vi "Init.vi"(8 "error in":errorcluster, 9 "IDNStr Override":string, 10 "Alias":string) -> (0 "error out":errorcluster, 3 "Instrument out":refnum<class "Instrument.lvclass">)   [LabVIEW 2014, in "Instrument.lvclass"]
uses:
  Instrument.lvclass
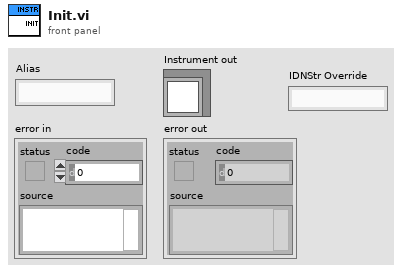
[diagram p1: front panel]
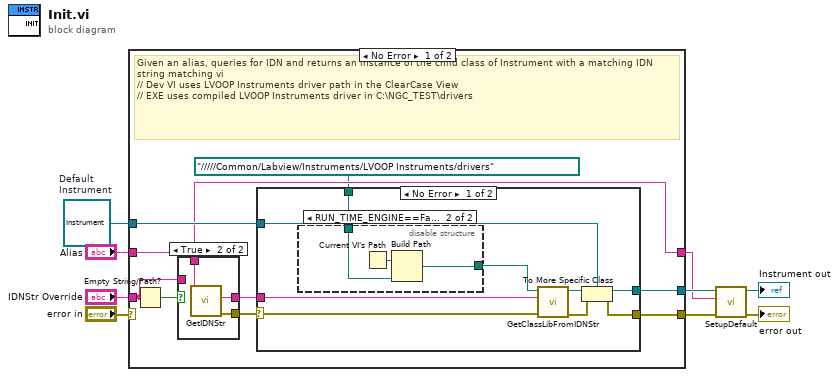
[diagram p0: block diagram]
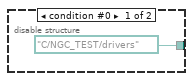
[diagram p3: hidden frame]
diagram:
  w7 = refnum<class "Instrument.lvclass"> refnum  # Default Instrument
  n1 = case shown="No Error" "error in" {
    selector: "error in" -> [_ w40]
    tunnel: "Alias" -> [w13 w38]
    tunnel: [w17 w39] -> w6
    tunnel: [w18 w40] -> w5
    tunnel: w7 -> [w14 w39]
    tunnel: [w13 w38] -> w2
    tunnel: "IDNStr Override" -> [w11 _]
    frame No Error {
      # "Given an alias, queries for IDN and returns an instance of the child class of Instrument with a matching IDN string matching vi\n// Dev VI uses LVOOP Instruments driver path in the ClearCase View\n// EXE uses compiled LVOOP Instruments driver in C:\\NGC_TEST\\drivers"
      n2 = Empty String/Path?(string/path=w11) -> (empty?=w12:bool)
      n3 = case shown="True" w12 {
        tunnel: [_ w22] -> w16
        tunnel: [w19 w21] -> w15
        tunnel: w13 -> [_ w20]
        tunnel: w11 -> [w19 _]
        frame False {
        }
        frame True {
          n4 = call "GetIDNStr.vi"("Alias"=w20) -> ("error out"=w22:errorcluster, "Model ID String"=w21:string)  [unwired: 9 in]
        }
      }
      n5 = case shown="No Error" w16 {
        selector: w16 -> [w30 w37]
        tunnel: [w27 w37] -> w18
        tunnel: [w25 w36] -> w17
        tunnel: w15 -> [w31 _]
        tunnel: w14 -> [w26 w36]
        tunnel: path "../../../../../Common/Labview/Instruments/LVOOP Instruments/drivers" -> [w24 _]
        frame No Error {
          n6 = disable-structure shown="RUN_TIME_ENGINE==False" {
            disable-tunnel: [path "C:/NGC_TEST/drivers" ("stripped path") w33] -> w23
            disable-tunnel: w24 -> [_ w35]
            frame condition #0 {
            }
            frame condition #1 (active) {
              n7 = Current VI's Path() -> (path=w34:path)
              n8 = Build Path(base path=w34, name or relative path=w35) -> (appended path=w33:path)
            }
          }
          n9 = call "GetClassLibFromIDNStr.vi"("error in"=w30, "IDNStr"=w31, "Driver folder"=w23) -> ("error out"=w28:errorcluster, "object"=w29:refnum<class>)  [unwired: 7 in]
          n10 = To More Specific Class(target class=w26, reference=w29, error in=w28) -> (specific class reference=w25:refnum<class "Instrument.lvclass">, error out=w27:errorcluster)
        }
        frame Error {
        }
      }
    }
    frame Error {
    }
  }
  n11 = call-dynamic "SetupDefault.vi"("error in (no error)"=w5, "Alias"=w2, "Instrument in"=w6) -> ("error out"=→"error out":errorcluster, "Instrument out"=→"Instrument out":refnum<class "Instrument.lvclass">)  [unwired: 7 in]
